vi "Inverse Kinematics.vi"(0 "v1":dbl[](array[numeric]), 1 "v2":dbl[](array[numeric]), 2 "v3":dbl[](array[numeric]), 3 "alpha1":dbl=0.7853981633974483, 4 "alpha2":dbl=0.7853981633974483, 5 "beta1":dbl=0.7853981633974483) -> (14 "theta":dbl[](array[numeric])=[1.5707963267948963, 1.570796326794896, 1.570796326794896])   [LabVIEW 2017]
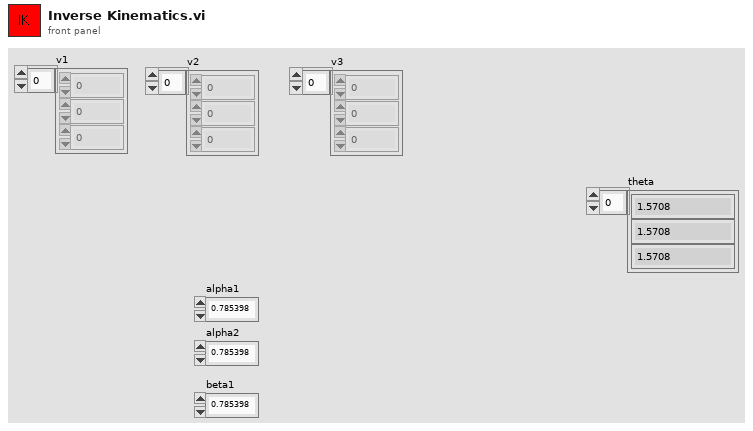
[diagram p1: front panel]
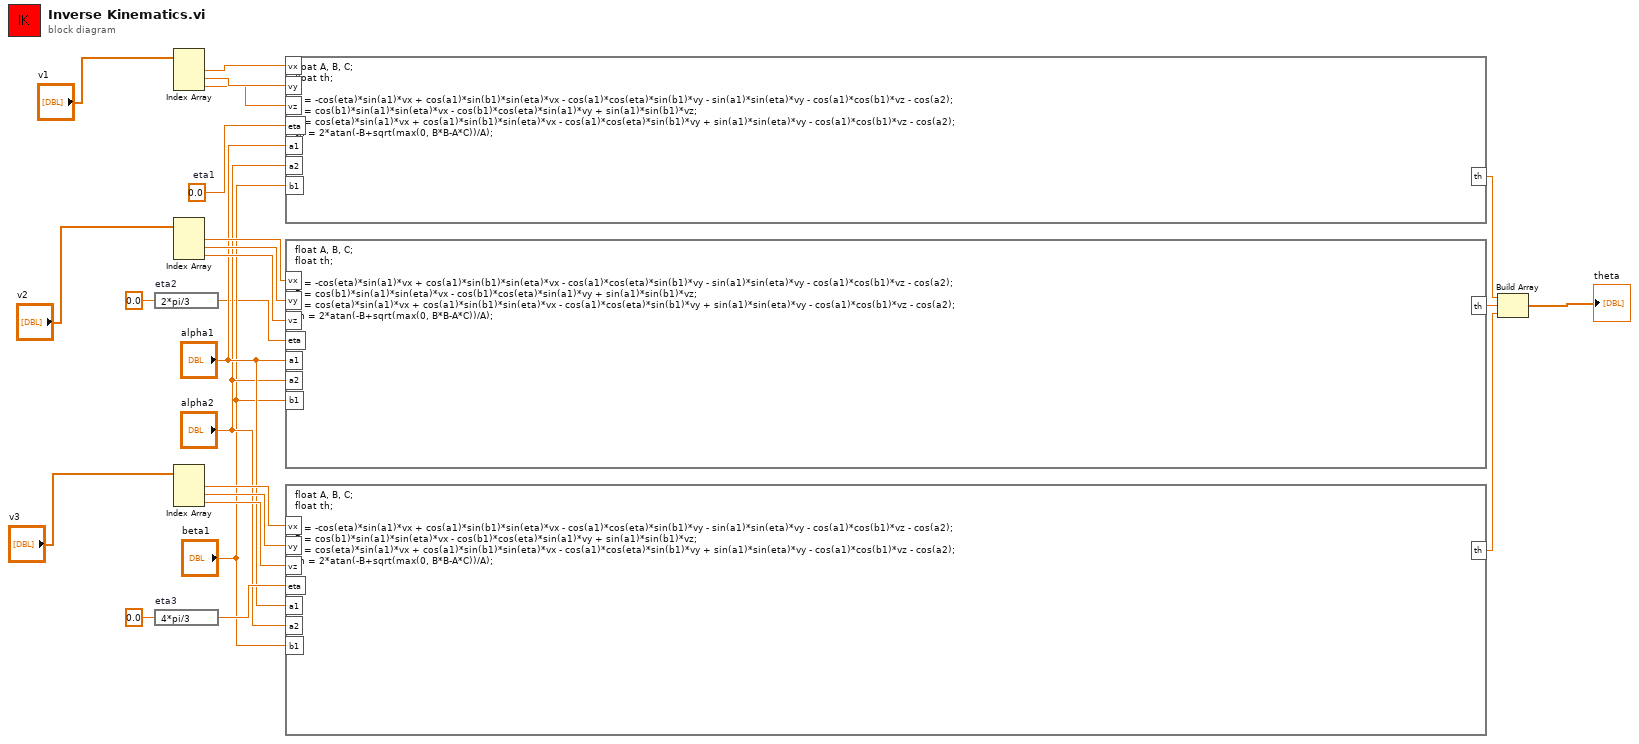
[diagram p0: block diagram]
diagram:
  w5 = 0.0  # eta1
  n1 = expression code="2*pi/3" "eta2"(0.0) -> (w6:dbl)
  n2 = expression code="4*pi/3" "eta3"(0.0) -> (w14:dbl)
  n3 = Index Array(array="v1") -> (element #1=w23:dbl, element #2=w22:dbl, element #3=w21:dbl)  [unwired: 3 in]
  n4 = Index Array(array="v2") -> (element #1=w20:dbl, element #2=w19:dbl, element #3=w18:dbl)  [unwired: 3 in]
  n5 = Index Array(array="v3") -> (element #1=w17:dbl, element #2=w16:dbl, element #3=w15:dbl)  [unwired: 3 in]
  n6 = formula code="float A, B, C;\nfloat th;\n\nA = -cos(eta)*sin(a1)*vx + cos(a1)*sin(b1)*sin(eta)*vx - cos(a1)*cos(eta)*sin(b1)*vy - sin(a1)*sin(eta)*vy - cos(a1)*cos(b1)*vz - cos(a2);\nB = cos(b1)*sin(a1)*sin(eta)*vx - cos(b1)*cos(eta)*sin(a1)*vy + sin(a1)*sin(b1)*vz;\nC = cos(eta)*sin(a1)*vx + cos(a1)*sin(b1)*sin(eta)*vx - cos(a1)*cos(eta)*sin(b1)*vy + sin(a1)*sin(eta)*vy - cos(a1)*cos(b1)*vz - cos(a2);\nth = 2*atan(-B+sqrt(max(0, B*B-A*C))/A);"("vx"=w23, "vy"=w22, "vz"=w21, "eta"=w5, "a1"="alpha1", "b1"="beta1", "a2"="alpha2") -> ("th"=w10:dbl)
  n7 = formula code="float A, B, C;\nfloat th;\n\nA = -cos(eta)*sin(a1)*vx + cos(a1)*sin(b1)*sin(eta)*vx - cos(a1)*cos(eta)*sin(b1)*vy - sin(a1)*sin(eta)*vy - cos(a1)*cos(b1)*vz - cos(a2);\nB = cos(b1)*sin(a1)*sin(eta)*vx - cos(b1)*cos(eta)*sin(a1)*vy + sin(a1)*sin(b1)*vz;\nC = cos(eta)*sin(a1)*vx + cos(a1)*sin(b1)*sin(eta)*vx - cos(a1)*cos(eta)*sin(b1)*vy + sin(a1)*sin(eta)*vy - cos(a1)*cos(b1)*vz - cos(a2);\nth = 2*atan(-B+sqrt(max(0, B*B-A*C))/A);"("vx"=w20, "vy"=w19, "vz"=w18, "eta"=w6, "a1"="alpha1", "b1"="beta1", "a2"="alpha2") -> ("th"=w9:dbl)
  n8 = formula code="float A, B, C;\nfloat th;\n\nA = -cos(eta)*sin(a1)*vx + cos(a1)*sin(b1)*sin(eta)*vx - cos(a1)*cos(eta)*sin(b1)*vy - sin(a1)*sin(eta)*vy - cos(a1)*cos(b1)*vz - cos(a2);\nB = cos(b1)*sin(a1)*sin(eta)*vx - cos(b1)*cos(eta)*sin(a1)*vy + sin(a1)*sin(b1)*vz;\nC = cos(eta)*sin(a1)*vx + cos(a1)*sin(b1)*sin(eta)*vx - cos(a1)*cos(eta)*sin(b1)*vy + sin(a1)*sin(eta)*vy - cos(a1)*cos(b1)*vz - cos(a2);\nth = 2*atan(-B+sqrt(max(0, B*B-A*C))/A);"("vx"=w17, "vy"=w16, "vz"=w15, "eta"=w14, "a1"="alpha1", "b1"="beta1", "a2"="alpha2") -> ("th"=w8:dbl)
  n9 = Build Array(w10, w9, w8) -> (→"theta":dbl[])
